vi "Set Images Path.vi"(8 "error in (no error)":errorcluster, 11 "ImageOperation in":refnum<class "ImageOperation.lvclass">) -> (0 "error out":errorcluster, 3 "ImageOperation out":refnum<class "ImageOperation.lvclass">)   [LabVIEW 2015, in "ImageOperation.lvclass"]
uses:
  ImageOperation.lvclass
  ImageOperation.lvclass/ImageOperation.ctl
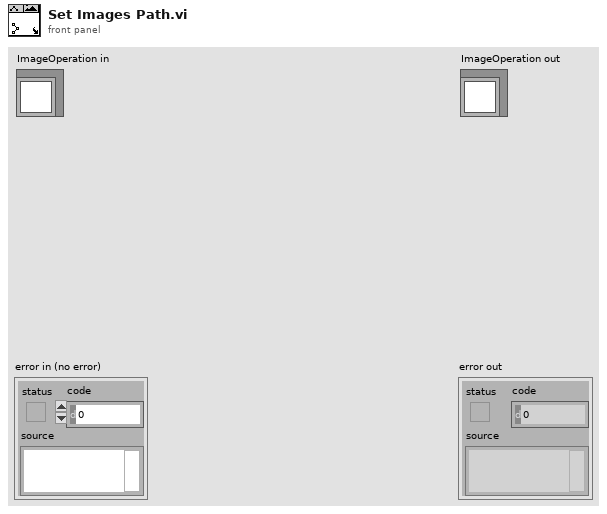
[diagram p1: front panel]
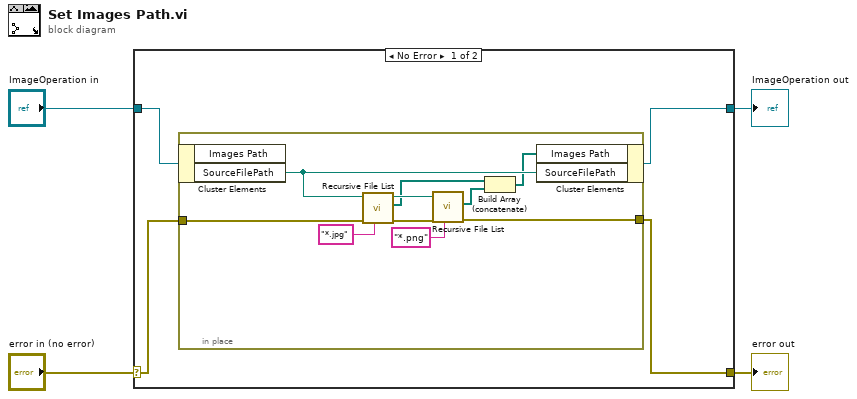
[diagram p0: block diagram]
diagram:
  n1 = case shown="No Error" "error in (no error)" {
    selector: "error in (no error)" -> [w7 w20]
    tunnel: [w5 w20] -> w3
    tunnel: [w6 w19] -> w1
    tunnel: "ImageOperation in" -> [w8 w19]
    frame No Error {
      n2 = in-place {
        in-place-border: w7 -> [w18]
        in-place-border: [w13] -> w5
        n3 = in-place-cluster #1(w8) -> ("SourceFilePath"=w17:path)  [unwired: 1 out]
        n4 = call <vilib>:"Recursive File List.vi"("pattern"="*.jpg", "error in (no error)"=w18, "Folder Path"=w17) -> ("error out"=w14:errorcluster, "All Files in Dir"=w11:path[], "dup Folder Path"=w15:path)  [unwired: 4 in, 2 out]
        n5 = call <vilib>:"Recursive File List.vi"("pattern"="*.png", "error in (no error)"=w14, "Folder Path"=w15) -> ("error out"=w13:errorcluster, "All Files in Dir"=w10:path[])  [unwired: 4 in, 3 out]
        n6 = Build Array (concatenate)(w11, w10) -> (w9:path[])
        n7 = in-place-cluster #1("Images Path"=w9, "SourceFilePath"=w17) -> (w6:refnum<class "ImageOperation.lvclass">)
      }
    }
    frame Error {
    }
  }
  "error out" <- w3
  "ImageOperation out" <- w1
